vi "timer_string.vi"(8 "error in (no error)":errorcluster, 10 "millisecond timer value":u32, 11 "millisecond timer value 2":u32) -> (0 "error out":errorcluster, 3 "String":string)   [LabVIEW 2017]
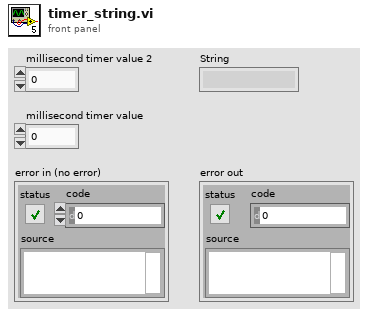
[diagram p1: front panel]
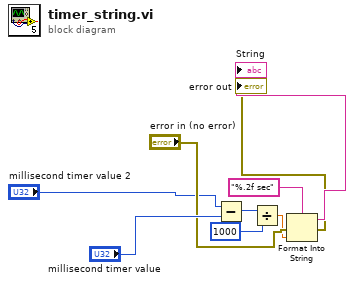
[diagram p0: block diagram]
diagram:
  n1 = Subtract(x="millisecond timer value 2", y="millisecond timer value") -> (x-y=w2:u32)
  n2 = Divide(x=w2, y=u32 1000) -> (x/y=w5:dbl)
  n3 = Format Into String(format string="%.2f sec", error in="error in (no error)", w5) -> (resulting string=→"String":string, error out=→"error out":errorcluster)  [unwired: 1 in]
